vi "Reset Sensors.vi"() -> ()   [LabVIEW 2014]
uses:
  <vilib>/Rock Robotics/WPI/PWM/WPI_PWMTransform_ConPane.ctl
  <vilib>/Rock Robotics/WPI/CAN/Jaguar/SubVIs/WPI_CANJaguar_ControlMode.ctl
  <vilib>/Rock Robotics/WPI/CAN/TalonSRX/WPI_CANTalonSRX_APIControlMode.ctl
  <vilib>/Rock Robotics/SystemInterfaces/Typedef/FPGA_TypedefDigitalModule.ctl
  <vilib>/Rock Robotics/SystemInterfaces/DIO/FPGA_DIOPWMChannel.ctl
  <vilib>/Rock Robotics/WPI/PWM/WPI_PWMDeadband.ctl
  <vilib>/Rock Robotics/WPI/MotorControl/WPI_MotorControlType.ctl
  <vilib>/Rock Robotics/WPI/MotorControl/WPI_MotorControlDeviceRef.ctl
  <vilib>/Rock Robotics/WPI/RobotDrive/WPI_RobotDriveDevRef.ctl
panel:
  in  "Drive Motors":T1={"DevStatus"={"status"=FALSE, "code"=0, "source"=""}, "Motors[]"=[], "Square Inputs"=FALSE, "Max Output"=1.0}
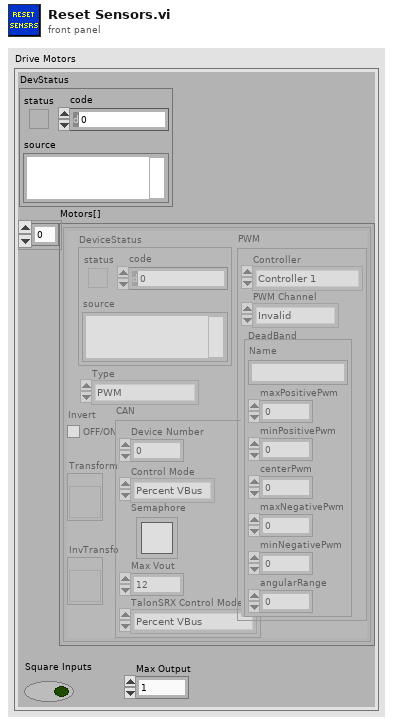
[diagram p1: front panel]
types:
  T1 = typedef "WPI_RobotDriveDevRef.ctl" = cluster{"DevStatus":errorcluster, "Motors[]":T2[], "Square Inputs":bool, "Max Output":dbl}
  T2 = typedef "WPI_MotorControlDeviceRef.ctl" = cluster{"DeviceStatus":errorcluster, "Type":T3, "PWM":cluster{"Controller":T4, "PWM Channel":T5, "DeadBand":T6}, "CAN":cluster{"Device Number":u8, "Control Mode":T7, "Semaphore":T8, "Max Vout":dbl, "TalonSRX Control Mode":T9}, "Invert":bool, "TransformRef":T10, "InvTransformRef":T10}
  T3 = typedef "WPI_MotorControlType.ctl" = enum16{"PWM", "CAN", "CANTalonSRX"}
  T4 = typedef "FPGA_TypedefDigitalModule.ctl" = enum16{"Controller 1"}
  T5 = typedef "FPGA_DIOPWMChannel.ctl" = enum8{"PWM 0", "PWM 1", "PWM 2", "PWM 3", "PWM 4", "PWM 5", "PWM 6", "PWM 7", "PWM 8", "PWM 9", "PWM MXP 0", "PWM MXP 1", "PWM MXP 2", "PWM MXP 3", "PWM MXP 4", "PWM MXP 5", "PWM MXP 6", "PWM MXP 7", "PWM MXP 8", "PWM MXP 9", "Invalid"}
  T6 = typedef "WPI_PWMDeadband.ctl" = cluster{"Name":string, "maxPositivePwm":i32, "minPositivePwm":i32, "centerPwm":i32, "maxNegativePwm":i32, "minNegativePwm":i32, "angularRange":u16}
  T7 = typedef "WPI_CANJaguar_ControlMode.ctl" = enum8{"Percent VBus", "Current", "Speed", "Position", "Voltage"}
  T8 = typedef "Semaphore RefNum" = refnum<k1>
  T9 = typedef "WPI_CANTalonSRX_APIControlMode.ctl" = enum8{"Percent VBus", "Speed", "Position", "Slave", "Unchanged / Invalid"}
  T10 = typedef "WPI_PWMTransform_ConPane.ctl" = refnum<vi>
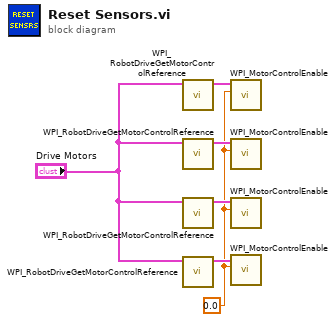
[diagram p0: block diagram]
diagram:
  w1 = 0.0 ("Encoder Initial Position")
  n1 = call <vilib>:"WPI_RobotDriveGetMotorControlReference.vi"("RobotDriveDevRef"="Drive Motors") -> ("MotorControlDeviceRef"=w5:T2)  [unwired: 1 in, 9 out]
  n2 = call <vilib>:"WPI_RobotDriveGetMotorControlReference.vi"("RobotDriveDevRef"="Drive Motors") -> ("MotorControlDeviceRef"=w4:T2)  [unwired: 1 in, 9 out]
  n3 = call <vilib>:"WPI_RobotDriveGetMotorControlReference.vi"("RobotDriveDevRef"="Drive Motors") -> ("MotorControlDeviceRef"=w3:T2)  [unwired: 1 in, 9 out]
  n4 = call <vilib>:"WPI_RobotDriveGetMotorControlReference.vi"("RobotDriveDevRef"="Drive Motors") -> ("MotorControlDeviceRef"=w2:T2)  [unwired: 1 in, 9 out]
  n5 = call <vilib>:"WPI_MotorControlEnable.vi"("Encoder Initial Position"=w1, "CAN Jaguar Ref"=w5) -> ()  [unwired: 8 in, 2 out]
  n6 = call <vilib>:"WPI_MotorControlEnable.vi"("Encoder Initial Position"=w1, "CAN Jaguar Ref"=w4) -> ()  [unwired: 8 in, 2 out]
  n7 = call <vilib>:"WPI_MotorControlEnable.vi"("Encoder Initial Position"=w1, "CAN Jaguar Ref"=w3) -> ()  [unwired: 8 in, 2 out]
  n8 = call <vilib>:"WPI_MotorControlEnable.vi"("Encoder Initial Position"=w1, "CAN Jaguar Ref"=w2) -> ()  [unwired: 8 in, 2 out]
